vi "Remove_FF_lone_spikes.vi"(3 "ADC Frequency Hz":dbl=1000.0 format="%.2f", 4 "Bkgnd variance":dbl format="%.6f", 5 "Analysis Info cluster":T1={"Colour"=0, "Inst type"=enum."Pitot-static tube", "Inst name"="Manometer voltage", "Symbol"="U", "Code name"="", "Extra Info"="U", "Inst Array"=enum."PWA", "Index"=0, "Voltage Index"=0, "Extra Titles"=[], "Extra Values"=[]}, 6 "Time Trace":dbl[](graph)) -> (0 "No Removed":i32, 1 "Analysis Info cluster out":T1={"Colour"=0, "Inst type"=enum."Pitot-static tube", "Inst name"="Manometer voltage", "Symbol"="U", "Code name"="", "Extra Info"="U", "Inst Array"=enum."PWA", "Index"=0, "Voltage Index"=0, "Extra Titles"=[], "Extra Values"=[]}, 2 "Filtered Time Trace":dbl[](graph))   [LabVIEW 2011]
uses:
  Controls/Analysis_info_cluster.ctl
  Controls/Inst_type.ctl
  Controls/Instrument_Array.ctl
  Globals/Meas_global.vi
  <vilib>/Analysis/NI_AALBase.lvlib
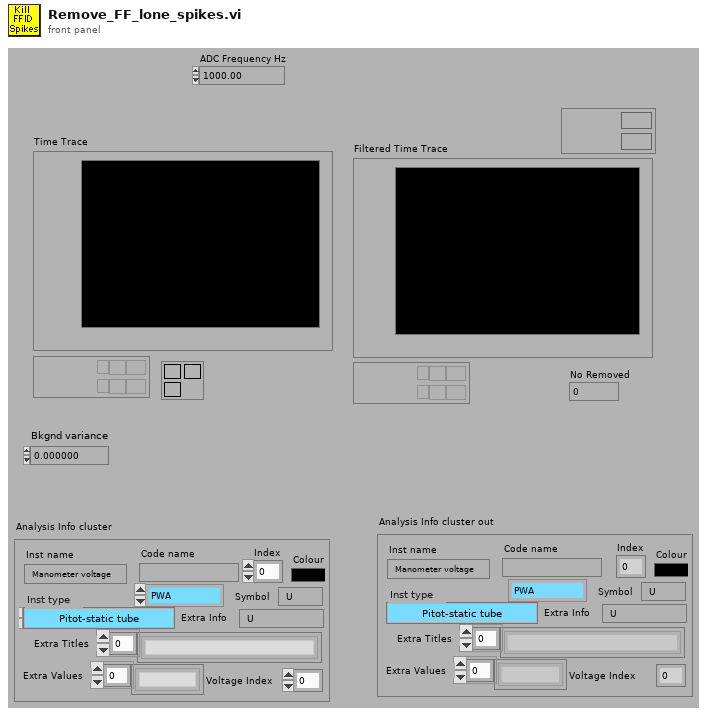
[diagram p1: front panel]
types:
  T1 = typedef "Analysis_info_cluster.ctl" = cluster{"Colour":u32, "Inst type":T2, "Inst name":string, "Symbol":string, "Code name":string, "Extra Info":string, "Inst Array":T3, "Index":i32, "Voltage Index":i32, "Extra Titles":string[], "Extra Values":string[]}
  T2 = typedef "Inst_type.ctl" = enum16{"Propeller anemometer", "Raw voltage", "Pressure Transducer", "Pitot-static tube", "Preston tube", "Hot wire", "Cross wire 1", "Cross wire 2", "Generic Linear", "Generic Polynomial", "Generic BackPoly", "Fast FID", "Thermocouple", "Cold wire", "Pulsed Wire", "LDA Vel", "LDA Tran time", "LDA Arr time"}
  T3 = typedef "Instrument_Array.ctl" = enum16{"PWA", "LDA", "Analogue"}
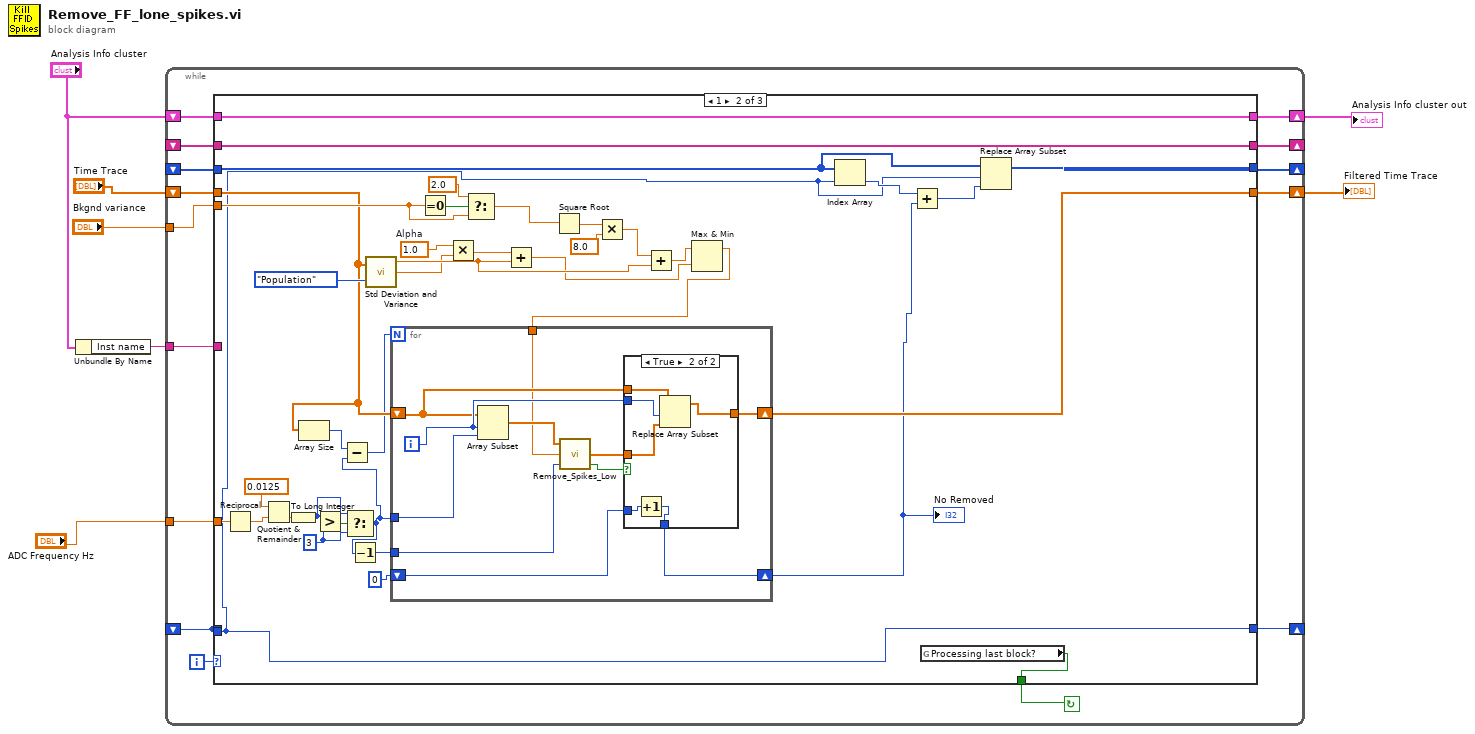
[diagram p0: block diagram]
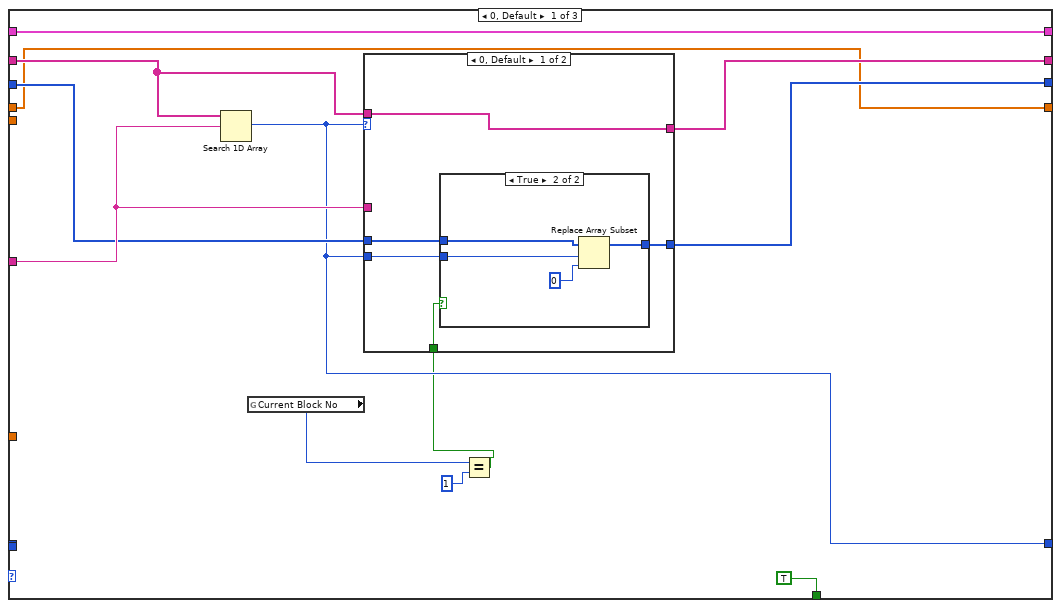
[diagram p2: hidden frame]
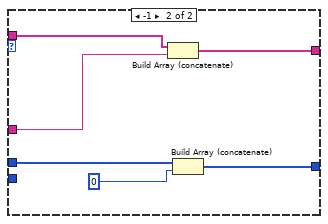
[diagram p4: hidden frame]
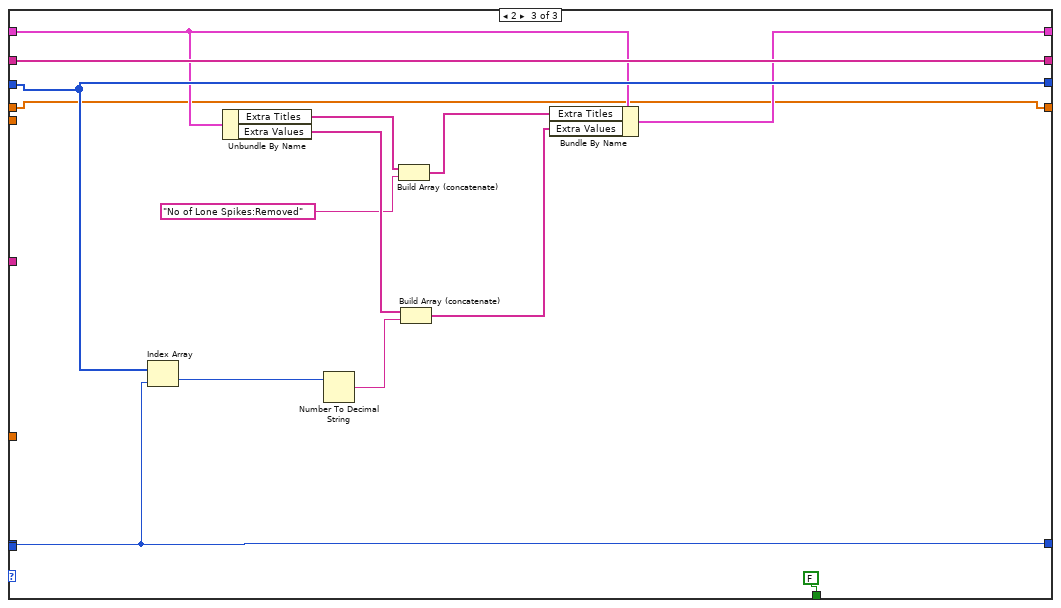
[diagram p6: hidden frame]
diagram:
  n1 = Unbundle By Name("Analysis Info cluster") -> ("Inst name"=w7:string)
  n2 = while {
    shift-left: _ -> [w19]
    shift-right: [w21] -> _
    tunnel: w7 -> [w18]
    shift-right: [w16] -> _
    shift-left: _ -> [w17]
    shift-right: [w14] -> _
    shift-left: _ -> [w15]
    shift-right: [w12] -> w5
    shift-left: "Analysis Info cluster" -> [w13]
    tunnel: "Bkgnd variance" -> [w11]
    shift-right: [w9] -> w2
    shift-left: "Time Trace" -> [w10]
    tunnel: "ADC Frequency Hz" -> [w8]
    i -> [w22]
    stop <- w20 continue-if-true
    n3 = case shown="1" w22 {
      tunnel: [w26 w59 w119] -> w21
      tunnel: [TRUE w57 FALSE ("Processing last block?")] -> w20
      tunnel: w19 -> [_ _ w119]
      tunnel: w19 -> [_ w59 _]
      tunnel: w18 -> [w30 _ _]
      tunnel: w17 -> [w31 w76 w117]
      tunnel: [w29 w76 w117] -> w16
      tunnel: w15 -> [w28 w75 w116]
      tunnel: [w27 w73 w116] -> w14
      tunnel: w13 -> [w24 w72 w113]
      tunnel: [w24 w72 w115] -> w12
      tunnel: w11 -> [_ w70 _]
      tunnel: w10 -> [w23 w63 w108]
      tunnel: [w23 w58 w108] -> w9
      tunnel: w8 -> [_ w68 _]
      frame 0, Default {
        n4 = Search 1D Array(1D array=w31, element=w30) -> (index of element=w26:i32)  [unwired: 1 out]
        n5 = global read "Meas_global.vi" "Current Block No"() -> (w33:i32)
        n6 = Equal?(x=w33, y=1) -> (x = y?=w25:bool)
        n7 = case shown="0, Default" w26 {
          tunnel: w31 -> [w39 w50]
          tunnel: w30 -> [_ w49]
          tunnel: [w39 w48] -> w29
          tunnel: w28 -> [w38 w47]
          tunnel: [w37 w46] -> w27
          tunnel: w26 -> [w36 _]
          tunnel: w25 -> [w35 _]
          frame 0, Default {
            n8 = case shown="True" w35 {
              tunnel: w38 -> [w40 w44]
              tunnel: [w40 w43] -> w37
              tunnel: w36 -> [_ w42]
              frame False {
              }
              frame True {
                n9 = Replace Array Subset(array=w44, new element=0, index=w42) -> (w43:i32[])
              }
            }
          }
          frame -1 {
            n10 = Build Array (concatenate)(w50, w49) -> (w48:string[])
            n11 = Build Array (concatenate)(w47, 0) -> (w46:i32[])
          }
        }
      }
      frame 1 {
        w53 = 3 ("y")
        w88 = 1.0  # Alpha
        n12 = Reciprocal(x=w68) -> (1/x=w66:dbl)
        n13 = Quotient & Remainder(x=0.0125, y=w66) -> (floor(x/y)=w65:dbl)  [unwired: 1 out]
        n14 = To Long Integer(number=w65) -> (32bit integer=w52:i32)
        n15 = Array Size(array=w63) -> (size(s)=w62:i32)
        n16 = Greater?(x=w52, y=w53) -> (0:w54:bool)
        n17 = Select(t=w52, s=w54, f=w53) -> (s? t:f=w51:i32)
        n18 = Subtract(x=w62, y=w51) -> (x-y=w61:i32)
        n19 = Decrement(x=w51) -> (x-1=w64:i32)
        n20 = call <vilib>:"Std Deviation and Variance.vi"("X"=w63, "Weighting (Sample)"=enum16{"Sample", "Population"}."Population") -> ("mean"=w83:dbl, "standard deviation"=w71:dbl)  [unwired: 1 out]
        n21 = Equal To 0?(x=w70) -> (x = 0?=w82:bool)
        n22 = Multiply(x=w88, y=w71) -> (x*y=w87:dbl)
        n23 = Select(t=2.0, s=w82, f=w70) -> (s? t:f=w80:dbl)
        n24 = Add(x=w87, y=w83) -> (x+y=w77:dbl)
        n25 = Square Root(x=w80) -> (sqrt(x)=w86:dbl)
        n26 = Multiply(x=w86, y=8.0) -> (x*y=w84:dbl)
        n27 = Add(x=w84, y=w83) -> (x+y=w78:dbl)
        n28 = Max & Min(x=w78, y=w77) -> (max(x,y)=w60:dbl)  [unwired: 1 out]
        n29 = for {
          N: w61 -> [_]
          shift-right: [w92] -> w58
          shift-left: w63 -> [w93]
          tunnel: w51 -> [w99]
          tunnel: w64 -> [w98]
          tunnel: w60 -> [w91]
          shift-right: [w90] -> w56
          shift-left: 0 -> [w89]
          i -> [w95]
          n30 = Array Subset(array=w93, index=w95, length=w99) -> (w97:dbl[])
          n31 = call "Remove_Spikes_Low.vi"("index"=w98, "Background noise"=w91, "Time Trace"=w97) -> ("Spike"=w96:bool, "Filtered Time Trace"=w94:dbl[])  [unwired: 1 out]
          n32 = case shown="True" w96 {
            tunnel: w95 -> [_ w107]
            tunnel: w94 -> [_ w106]
            tunnel: w93 -> [w101 w105]
            tunnel: [w101 w104] -> w92
            tunnel: [w100 w102] -> w90
            tunnel: w89 -> [w100 w103]
            frame False {
            }
            frame True {
              n33 = Increment(x=w103) -> (x+1=w102:i32)
              n34 = Replace Array Subset(array=w105, new element=w106, index=w107) -> (w104:dbl[])
            }
          }
        }
        "No Removed" <- w56
        n35 = Index Array(array=w75, index=w59) -> (element=w74:i32)
        n36 = Add(x=w74, y=w56) -> (x+y=w69:i32)
        n37 = global read "Meas_global.vi" "Processing last block?"() -> (w57:bool)
        n38 = Replace Array Subset(array=w75, new element=w69, index=w59) -> (w73:i32[])
      }
      frame 2 {
        n39 = Index Array(array=w116, index=w119) -> (element=w118:i32)
        n40 = Unbundle By Name(w113) -> ("Extra Titles"=w112:string[], "Extra Values"=w111:string[])
        n41 = Number To Decimal String(number=w118) -> (decimal integer string=w120:string)  [unwired: 1 out]
        n42 = Build Array (concatenate)(w112, "No of Lone Spikes:Removed" ("format string")) -> (w114:string[])
        n43 = Build Array (concatenate)(w111, w120) -> (w110:string[])
        n44 = Bundle By Name(cluster=w113, "Extra Titles"=w114, "Extra Values"=w110) -> (w115:T1)
      }
    }
  }
  "Analysis Info cluster out" <- w5
  "Filtered Time Trace" <- w2
